vi "Main.vi"() -> ()   [LabVIEW 2020, in "PicoG-Processor.lvlib"]
uses:
  PicoG-Processor.lvlib
  GVIWebProcessorApp/GVIWebProcessorApp.lvclass
panel:
  out "error out":errorcluster
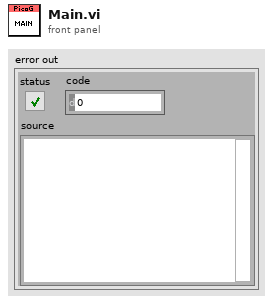
[diagram p1: front panel]
types:
  T1 = enum32{"Invalid", "Standard", "Closed", "Hidden", "Minimized", "Maximized"}
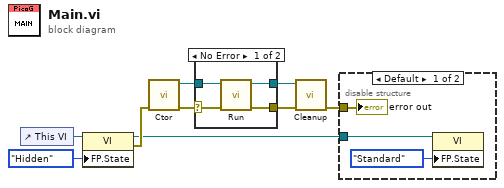
[diagram p0: block diagram]
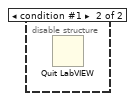
[diagram p2: hidden frame]
diagram:
  n1 = control-ref of="This VI"() -> (w9:refnum<vi>)
  n2 = property class="VI"(reference=w9, "FP.State"=T1."Hidden" ("Front Panel Window:State")) -> (reference out=w2:refnum<vi>, error out=w7:errorcluster)  [unwired: 1 in]
  n3 = call "Ctor.vi"("error in (no error)"=w7) -> ("error out"=w6:errorcluster, "GVIWebProcessorApp out"=w5:refnum<class "GVIWebProcessorApp.lvclass">)  [unwired: 9 in]
  n4 = case shown="No Error" w6 {
    selector: w6 -> [w12 w14]
    tunnel: w5 -> [w13 w15]
    tunnel: [w11 w15] -> w4
    tunnel: [w10 w14] -> w3
    frame No Error {
      n5 = call "Run.vi"("error in (no error)"=w12, "GVIWebProcessorApp in"=w13) -> ("error out"=w10:errorcluster, "GVIWebProcessorApp out"=w11:refnum<class "GVIWebProcessorApp.lvclass">)  [unwired: 8 in]
    }
    frame Error {
    }
  }
  n6 = call "Cleanup.vi"("error in (no error)"=w3, "GVIWebProcessorApp in"=w4) -> ("error out"=w1:errorcluster)  [unwired: 9 in]
  n7 = disable-structure shown="Default" {
    disable-tunnel: w2 -> [w17 _]
    disable-tunnel: w1 -> [w16 _]
    frame condition #0 (active) {
      n8 = property class="VI"(reference=w17, "FP.State"=T1."Standard" ("Front Panel Window:State")) -> ()  [unwired: 1 in, 2 out]
      "error out" <- w16
    }
    frame condition #1 {
      n9 = Quit LabVIEW() -> ()  [unwired: 1 in]
    }
  }
